vi "Log Event.vi"(8 "error in":errorcluster, 10 "Event Text":string, 11 "Series UI Actor in":refnum<class "Series UI Actor.lvclass">) -> (0 "error out":errorcluster, 3 "Series UI Actor out":refnum<class "Series UI Actor.lvclass">)   [LabVIEW 2024, in "Series UI Actor.lvlib" / "Series UI Actor.lvclass"]
uses:
  Series UI Actor.lvclass
  Series UI Actor.lvclass/Series UI Actor.ctl
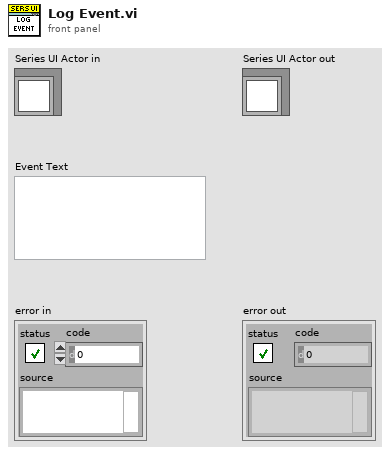
[diagram p1: front panel]
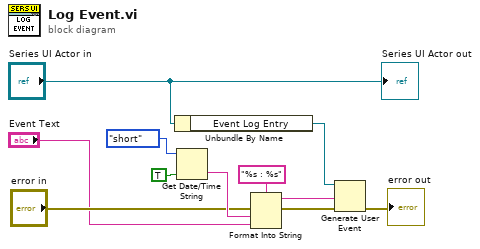
[diagram p0: block diagram]
diagram:
  n1 = Unbundle By Name("Series UI Actor in") -> ("Event Log Entry"=w11:refnum<user-event>)
  n2 = Get Date/Time String(date format (0)=enum16{"short", "long", "abbreviated"}."short", want seconds? (F)=TRUE) -> (time string=w8:string)  [unwired: 1 in, 1 out]
  n3 = Format Into String(format string="%s : %s", error in="error in", w8, "Event Text") -> (resulting string=w7:string, error out=w4:errorcluster)  [unwired: 1 in]
  n4 = Generate User Event(user event=w11, event data cluster=w7, error in=w4) -> (error out=→"error out":errorcluster)  [unwired: 1 in, 1 out]
  "Series UI Actor out" <- "Series UI Actor in"
